vi "tool_Unicode_Update String Control.vi"(9 "error in (no error)":errorcluster, 10 "String (UTF-16)":string, 11 "*StrControl in":refnum<vi>) -> (1 "error out":errorcluster, 3 "*StrControl out":refnum<vi>)   [LabVIEW 2013, in "SET_Unicode Tools.lvlib"]
doc: "tool_Unicode_Update String Control.vi\n\nUpdate a unicode string control's value by ref."
uses:
  SET_Unicode Tools.lvlib
panel:
  # "tool_Unicode_Update String Control.vi\n\nUpdate a unicode string control's value by ref."
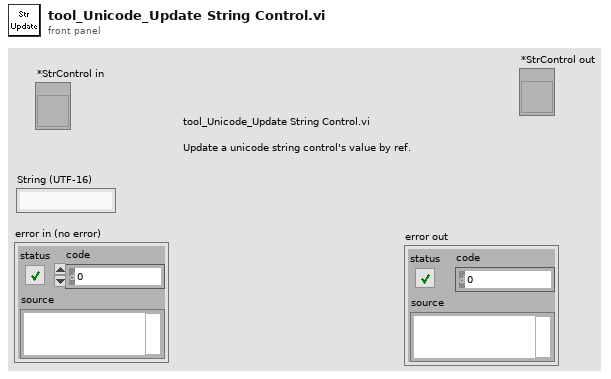
[diagram p1: front panel]
types:
  T1 = typedef "LVSelectionTypeDef.ctl" = cluster{"Selection Start":u32, "Selection End":u32}
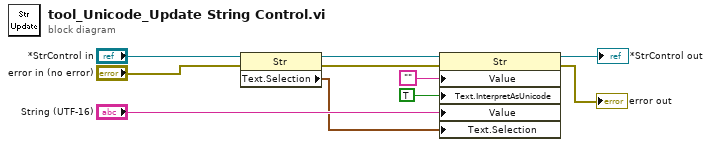
[diagram p0: block diagram]
diagram:
  n1 = property class="Str"(reference="*StrControl in", error in="error in (no error)") -> (reference out=w10:refnum<vi>, error out=w6:errorcluster, "Text.Selection"=w1:T1)
  n2 = property class="Str"(reference=w10, error in=w6, "Value"="", "Text.InterpretAsUnicode"=TRUE ("Text.Interpret As Unicode"), "Value"="String (UTF-16)", "Text.Selection"=w1) -> (reference out=→"*StrControl out":refnum<vi>, error out=→"error out":errorcluster)
